vi "MainLoop.vi"() -> ()   [LabVIEW 2021]
uses:
  <vilib>/Platform/TimedLoop/XDataNode/timing_clust.ctl
  <vilib>/Platform/TimedLoop/XDataNode/nitl_modes.ctl
  <vilib>/Platform/TimedLoop/XDataNode/wakeup.ctl
  <vilib>/DAQmx/write.llb/DAQmx Write (Analog 1D DBL NChan 1Samp).vi
  <vilib>/DAQmx/read.llb/DAQmx Read (Analog 1D DBL NChan 1Samp).vi
  5a09477c-fa6a-4a2c-ae4e-0462b0b96a3d.vi
  6f825153-6f78-4197-a3b4-cb3bcc6ce098.vi
  <vilib>/DAQmx/create/channels.llb/DAQmx Create Channel (AO-Voltage-Basic).vi
  <vilib>/DAQmx/create/channels.llb/DAQmx Create Channel (AI-Voltage-Basic).vi
  GlobalSTATE.vi
  <vilib>/DAQmx/miscellaneous.llb/DAQmx Fill In Error Info.vi
  Global_BeamBreaks.vi
  <vilib>/Utility/file.llb/Write Delimited Spreadsheet (string).vi
  <vilib>/Utility/file.llb/Read Delimited Spreadsheet (DBL).vi
  <vilib>/platform/TimedLoop/XDataNode/XDataNode.xnode
  <vilib>/Platform/TimedLoop/XDataNode/XDNodeRunTimeDep.lvlib
panel:
  out "ConditionVoltage":dbl
  out "BeamVoltage":dbl
  in  "stop":bool
  in  "Tab Control":enum32{"Settings", "Monitor", "Events"}(tab)
  in  "Task type":T1(ring)
  in  "Drive to change (in 'One drive changes')":enum32{"Food", "Water", "Social"}(ring)
  in  "Possible availability":i32[](array[numeric])=[0, 1, 2]
  in  "Control availability":i32=1
  in  "Availability settings":i32[][](array[numeric])=[[0, 1, 3], [0, 1, 3], [0, 3000, 9000]]
  in  "file (use dialog)":path=path "C:/Code/Availability-maze-main/Availability-maze-main/MazeCode/LookUpTbl.txt"
  in  "thresholds":dbl[](array[numeric])=[3.0, 2.0, 2.0, 2.0, 2.0, 2.0]
  in  "Beam breaks":bool[](array[boolean])
  out "Current State":string="Condition: l - 210"
  out "Block length":i32=3
  out "Max pellets":u32=2
  out "Interaction time (ms)":u32
  out "Max water drops":u32=1
  out "Block count":i32
  out "Trial of block":i32
  out "Food available":dbl(knob)=2.0 scale=0.0..3.0
  out "Water available":dbl(knob)=1.0 scale=0.0..3.0
  out "Social time available":dbl(knob) scale=0.0..10000.0
  out "serial comm":string="l"
  out "ms in nest":i32
  out "NEST":bool=TRUE
  out "Event times":string[][](array[string])=[["05/06/2022", "14:41:05", "SOCIAL TIME"], ["05/06/2022", "14:41:05", "Condition: l - 210"]]
  in  "Save event file?":bool
  in  "file path (dialog if empty)":path=path "C:/temp/EventData/222"
  # "Social\n\nWater\n\nFood\n\nMiddle 1\n\nMiddle 2\n\nHome cage"
  # "Low (0)     Medium (1)    High(2)"
  # "Pellets \n\nWater drops\n\nSocial time (ms)"
  # "This should stay at 1"
  # "Social                Water                  Food               Middle            Middle 2       Home cage"
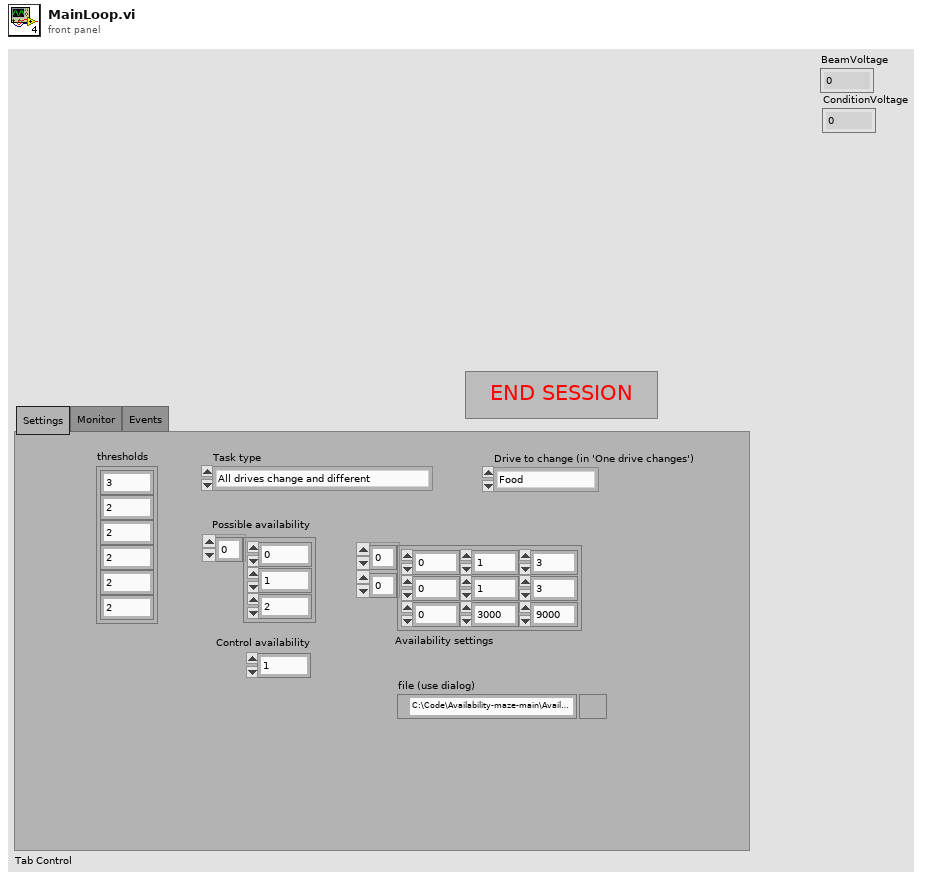
[diagram p1: front panel]
types:
  T1 = enum32{"All drives change and different", "One drive changes", "All drives same, but change"}
  T2 = typedef "XDNodeRunTimeDep.lvlib/timing_clust.ctl" = cluster{"Expected End [f-1]":u64, "Actual End [f-1]":u64, "Finished Late? [f-1]":bool, "Expected End [i-1]":u64, "Actual End [i-1]":u64, "Finished Late? [i-1]":bool, "Expected Start [i]":u64, "Actual Start [i]":u64, "Expected Start [f]":u64, "Actual Start [f]":u64, "Source Name":string, "Structure Name":string, "Period":i64, "Deadline":i64, "Offset":i64, "Start":i64, "Priority":i32, "Timeout":i32, "Mode":T3, "Wakeup Reason":T4, "Error":errorcluster, "Source Type":string, "Secondary Source Type":string, "Global End Time":u64, "Global Start Time":u64, "Frame Duration":u64, "Iteration Duration":u64, "Assigned CPU":i32, "I/O Scan Engine Mode":u32}
  T3 = typedef "XDNodeRunTimeDep.lvlib/nitl_modes.ctl" = enum32{"No Change", "Process missed periods, maintain original phase", "Discard missed periods, maintain original phase", "Process missed periods, ignore original phase", "Discard missed periods, ignore original phase"}
  T4 = typedef "XDNodeRunTimeDep.lvlib/wakeup.ctl" = enum32{"Normal", "Aborted", "Asynchronous wakeup", "Timing source error", "Timed loop error", "Timeout"}
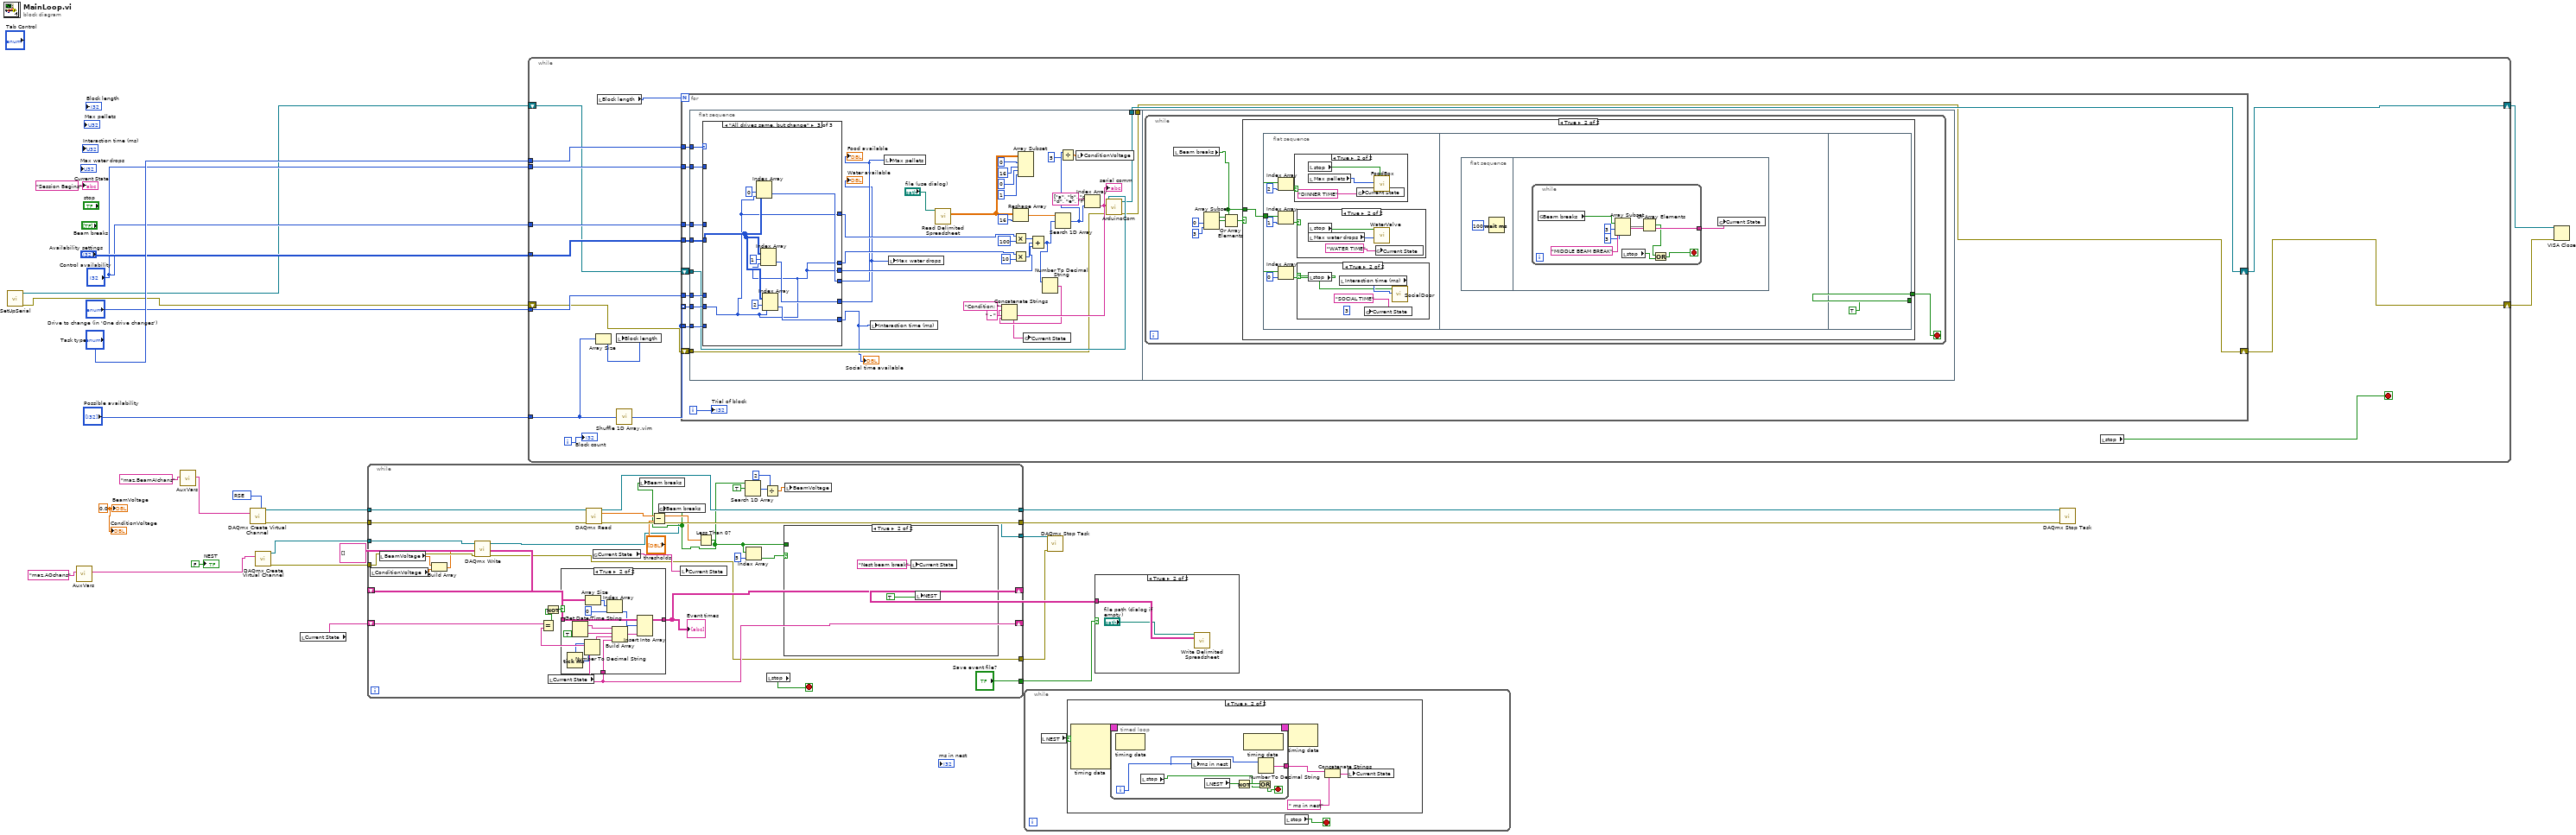
[diagram p0: block diagram]
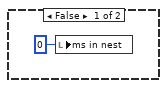
[diagram p2: hidden frame]
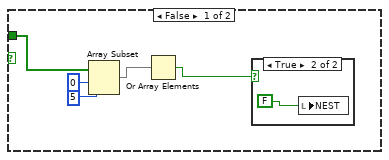
[diagram p4: hidden frame]
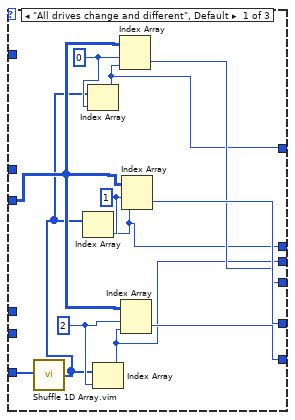
[diagram p7: hidden frame]
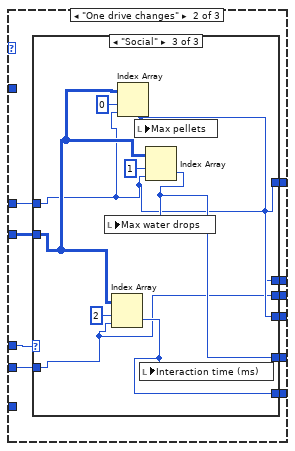
[diagram p8: hidden frame]
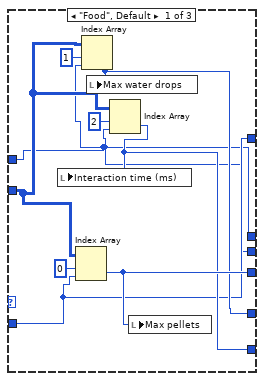
[diagram p9: hidden frame]
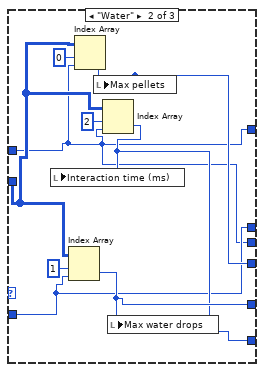
[diagram p10: hidden frame]
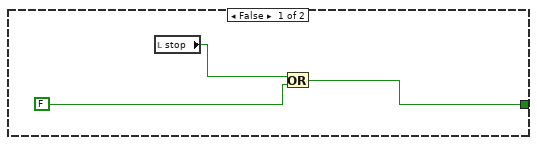
[diagram p11: hidden frame]
diagram:
  w9 = 0.0 ("BeamVoltage")
  w14 = 10083 items=["Default"=-1, "RSE"=10083, "NRSE"=10078, "Differential"=10106, "Pseudodifferential"=12529] ("input terminal configuration")
  n1 = call "SetUpSerial.vi"() -> ("error out"=w1:errorcluster, "VISA resource name out"=w16:refnum<visa-resource-name>)  [unwired: 10 in]
  n2 = call "AuxVars.vi"("key"="maz.AOchans") -> ("value"=w5:string)  [unwired: 9 in, 1 out]
  n3 = call "AuxVars.vi"("key"="maz.BeamAIchans") -> ("value"=w3:string)  [unwired: 9 in, 1 out]
  n4 = call-poly <vilib>:"DAQmx Create Virtual Channel.vi"("input terminal configuration"=w14, "physical channels"=w3) -> ("task out"=w29:refnum<k21>, "error out"=w28:errorcluster)  [unwired: 12 in]
  n5 = call-poly <vilib>:"DAQmx Create Virtual Channel.vi"("physical channels"=w5) -> ("task out"=w11:refnum<k21>, "error out"=w10:errorcluster)  [unwired: 13 in]
  n6 = local read "Current State"() -> (w18:string)
  n7 = while {
    tunnel: w29 -> [w59]
    tunnel: w28 -> [w58]
    tunnel: [w57] -> w27
    tunnel: [w56] -> w26
    shift-right: [w51] -> w17
    shift-left: string[][] [] -> [w52]
    shift-right: [w50] -> _
    shift-left: w18 -> [w49]
    tunnel: ["Save event file?"] -> w13
    tunnel: w11 -> [w41]
    tunnel: w10 -> [w40]
    tunnel: [w31] -> w8
    tunnel: [w30] -> w7
    stop <- w55 stop-if-true
    n8 = local read "ConditionVoltage"() -> (w33:dbl)
    n9 = local read "BeamVoltage"() -> (w34:dbl)
    n10 = Build Array(w34, w33) -> (w32:dbl[])
    n11 = call-poly <vilib>:"DAQmx Write.vi"("task/channels in"=w41, "data"=w32, "error in"=w40) -> ("task out"=w31:refnum<k21>, "error out"=w30:errorcluster)  [unwired: 10 in, 1 out]
    n12 = local read "Current State"() -> (w50:string)
    n13 = Equal?(x=w49, y=w50) -> (x = y?=w53:bool)
    n14 = Not(x=w53) -> (.not. x?=w54:bool)
    n15 = case shown="True" w54 {
      tunnel: w52 -> [w68 w80]
      tunnel: [w68 w79] -> w51
      tunnel: w50 -> [_ w74]
      frame False {
      }
      frame True {
        n16 = Tick Count (ms)() -> (millisecond timer value=w69:u32)
        n17 = Get Date/Time String(want seconds? (F)=TRUE) -> (date string=w73:string, time string=w71:string)  [unwired: 2 in]
        n18 = Number To Decimal String(number=w69, width (-)=w69) -> (decimal integer string=w70:string)
        n19 = Array Size(array=w80) -> (size(s)=w78:i32[])
        n20 = Index Array(array=w78, index=0) -> (element=w76:i32)
        n21 = Build Array(w73, w71, w70, w74) -> (w75:string[])
        n22 = Insert Into Array(array=w80, index (row)=w76, new element=w75) -> (w79:string[][])  [unwired: 1 in]
      }
    }
    "Event times" <- w51
    n23 = call-poly <vilib>:"DAQmx Read.vi"("task/channels in"=w59, "error in"=w58) -> ("task out"=w57:refnum<k21>, "data"=w46:dbl[], "error out"=w56:errorcluster)  [unwired: 11 in]
    n24 = global read "GlobalSTATE.vi" "Current State"() -> (w48:string)
    n25 = Subtract(x=w46, y="thresholds") -> (x-y=w47:dbl[])
    n26 = local write "Current State"(w48) -> ()
    n27 = Less Than 0?(x=w47) -> (x < 0?=w36:bool[])
    n28 = local write "Beam breaks"(w36) -> ()
    n29 = global write "Global_BeamBreaks.vi" "Beam breaks"(w36) -> ()
    n30 = Search 1D Array(1D array=w36, element=TRUE) -> (index of element=w39:i32)  [unwired: 1 in]
    n31 = Index Array(array=w36, index=5) -> (element=w43:bool)
    n32 = Divide(x=w39, y=2) -> (x/y=w37:dbl)
    n33 = local read "stop"() -> (w55:bool)
    n34 = case shown="True" w43 {
      tunnel: w36 -> [w64 _]
      frame False {
        n35 = Array Subset(array=w64, index=0, length=5) -> (w61:bool[])
        n36 = Or Array Elements(Boolean array=w61) -> (logical OR=w60:bool)
        n37 = case shown="True" w60 {
          frame False {
          }
          frame True {
            n38 = local write "NEST"(FALSE) -> ()
          }
        }
      }
      frame True {
        n39 = local write "Current State"("Nest beam break" ("Current State")) -> ()
        n40 = local write "NEST"(TRUE) -> ()
      }
    }
    n41 = local write "BeamVoltage"(w37) -> ()
  }
  n42 = while {
    tunnel: "Task type" -> [w95]
    tunnel: "Drive to change (in 'One drive changes')" -> [w94]
    tunnel: "Possible availability" -> [w89]
    tunnel: "Availability settings" -> [w93]
    tunnel: "Control availability" -> [w92]
    tunnel: "Control availability" -> [w91]
    shift-right: [w82] -> w2
    shift-left: w16 -> [w84]
    shift-right: [w81] -> w15
    shift-left: w1 -> [w83]
    i -> [w87]
    stop <- w85 stop-if-true
    n43 = Array Size(array=w89) -> (size(s)=w88:i32)
    n44 = local read "Block length"() -> (w90:i32)
    n45 = local write "Block length"(w88) -> ()
    n46 = call "Shuffle 1D Array.vim"("array"=w89) -> ("shuffled array"=w86:i32[])  [unwired: 4 in]
    n47 = for {
      N: w90 -> [_]
      tunnel: w95 -> [w107]
      tunnel: w94 -> [w106]
      tunnel: w86 -> [w105] mode=indexing
      tunnel: w93 -> [w104]
      tunnel: w92 -> [w103]
      tunnel: w91 -> [w102]
      tunnel: w86 -> [w100]
      shift-right: [w97] -> w82
      shift-left: w84 -> [w99]
      shift-right: [w96] -> w81
      shift-left: w83 -> [w98]
      i -> [w101]
      n48 = flat-sequence {
        tunnel: w107 -> [w146]
        tunnel: w106 -> [w145]
        tunnel: w105 -> [w144]
        tunnel: w104 -> [w143]
        tunnel: w103 -> [w142]
        tunnel: w102 -> [w141]
        tunnel: w100 -> [w140]
        tunnel: w99 -> [w117]
        tunnel: w98 -> [w116]
        tunnel: [w115] -> w97
        tunnel: [w114] -> w96
        frame #0 {
          n49 = case shown="\"All drives same, but change\"" w146 {
            tunnel: w145 -> [_ w168 _]
            tunnel: w144 -> [_ w167 w196]
            tunnel: w143 -> [w158 w166 w200]
            tunnel: w142 -> [_ _ _]
            tunnel: w141 -> [_ w165 _]
            tunnel: [w150 w164 w199] -> w112
            tunnel: [w151 w163 w198] -> w111
            tunnel: [w155 w162 w197] -> w113
            tunnel: w140 -> [w157 _ _]
            tunnel: [w149 w161 w196] -> w137
            tunnel: [w148 w160 w196] -> w136
            tunnel: [w147 w159 w196] -> w135
            frame "All drives change and different", Default {
              w154 = 0 ("index")
              w153 = 1 ("index")
              w156 = 2 ("index")
              n50 = call "Shuffle 1D Array.vim"("array"=w157) -> ("shuffled array"=w152:i32[])  [unwired: 4 in]
              n51 = Index Array(array=w152, index=w153) -> (element=w148:i32)
              n52 = Index Array(array=w152, index=w154) -> (element=w149:i32)
              n53 = Index Array(array=w152, index=w156) -> (element=w147:i32)
              n54 = Index Array(array=w158, index (row)=w154, index (col)=w149) -> (element=w150:i32)
              n55 = Index Array(array=w158, index (row)=w156, index (col)=w147) -> (element=w155:i32)
              n56 = Index Array(array=w158, index (row)=w153, index (col)=w148) -> (element=w151:i32)
            }
            frame "One drive changes" {
              n57 = case shown="\"Social\"" w168 {
                tunnel: w167 -> [w170 w179 w187]
                tunnel: w166 -> [w174 w183 w192]
                tunnel: w165 -> [w169 w178 w188]
                tunnel: [w173 w182 w189] -> w164
                tunnel: [w172 w181 w191] -> w163
                tunnel: [w171 w180 w190] -> w162
                tunnel: [w170 w178 w188] -> w161
                tunnel: [w169 w179 w188] -> w160
                tunnel: [w169 w178 w187] -> w159
                frame "Food", Default {
                  n58 = Index Array(array=w174, index (row)=0 ("index"), index (col)=w170) -> (element=w173:i32)
                  n59 = Index Array(array=w174, index (row)=1, index (col)=w169) -> (element=w172:i32)
                  n60 = local write "Max water drops"(w172) -> ()
                  n61 = Index Array(array=w174, index (row)=2 ("disabled index (row)"), index (col)=w169) -> (element=w171:i32)
                  n62 = local write "Interaction time (ms)"(w171) -> ()
                  n63 = local write "Max pellets"(w173) -> ()
                }
                frame "Water" {
                  n64 = Index Array(array=w183, index (row)=1 ("index"), index (col)=w179) -> (element=w181:i32)
                  n65 = Index Array(array=w183, index (row)=0, index (col)=w178) -> (element=w182:i32)
                  n66 = local write "Max pellets"(w182) -> ()
                  n67 = Index Array(array=w183, index (row)=2 ("disabled index (row)"), index (col)=w178) -> (element=w180:i32)
                  n68 = local write "Interaction time (ms)"(w180) -> ()
                  n69 = local write "Max water drops"(w181) -> ()
                }
                frame "Social" {
                  n70 = Index Array(array=w192, index (row)=2 ("index"), index (col)=w187) -> (element=w190:i32)
                  n71 = Index Array(array=w192, index (row)=0, index (col)=w188) -> (element=w189:i32)
                  n72 = local write "Max pellets"(w189) -> ()
                  n73 = local write "Interaction time (ms)"(w190) -> ()
                  n74 = Index Array(array=w192, index (row)=1 ("disabled index (row)"), index (col)=w188) -> (element=w191:i32)
                  n75 = local write "Max water drops"(w191) -> ()
                }
              }
            }
            frame "All drives same, but change" {
              n76 = Index Array(array=w200, index (row)=0, index (col)=w196) -> (element=w199:i32)
              n77 = Index Array(array=w200, index (row)=1, index (col)=w196) -> (element=w198:i32)
              n78 = Index Array(array=w200, index (row)=2, index (col)=w196) -> (element=w197:i32)
            }
          }
          "Food available" <- w112
          "Water available" <- w111
          "Social time available" <- w113
          n79 = local write "Interaction time (ms)"(w113) -> ()
          n80 = local write "Max pellets"(w112) -> ()
          n81 = local write "Max water drops"(w111) -> ()
          n82 = call-poly <vilib>:"Read Delimited Spreadsheet.vi"("file path (dialog if empty)"="file (use dialog)") -> ("all rows"=w127:dbl[][])  [unwired: 9 in, 5 out]
          n83 = Reshape Array(w127, 16 ("dimension size")) -> (w126:dbl[])
          n84 = Multiply(x=w137, y=100) -> (x*y=w133:i32)
          n85 = Multiply(x=w136, y=10) -> (x*y=w134:i32)
          n86 = Array Subset(array=w127, index (row)=0 ("index"), length (row)=16 ("length"), index (col)=0 ("index"), length (col)=1 ("length")) -> ()  [unwired: 1 out]
          n87 = Compound Arithmetic op=ADD(w133, w134, w135) -> (w120:i32)
          n88 = Number To Decimal String(number=w120) -> (decimal integer string=w119:string)  [unwired: 1 in]
          n89 = Search 1D Array(1D array=w126, element=w120) -> (index of element=w109:i32)  [unwired: 1 in]
          n90 = Divide(x=w109, y=5) -> (x/y=w110:dbl)
          n91 = local write "ConditionVoltage"(w110) -> ()
          n92 = Index Array(array=string[] ["a", "b", "c", "d", "e", "f", "g", "h", "i", "j", "k", "l", "m", "n", "o"], index=w109) -> (element=w122:string)
          "serial comm" <- w122
          n93 = Concatenate Strings("Condition: " ("string"), w122, " - " ("string"), w119) -> (w118:string)
          n94 = global write "GlobalSTATE.vi" "Current State"(w118) -> ()
          n95 = call "ArduinoCom.vi"("error out"=w116, "write buffer"=w122, "VISA resource name out"=w117) -> ("error out 2"=w114:errorcluster, "VISA resource name out 2"=w115:refnum<visa-resource-name>)  [unwired: 7 in]
        }
        frame #1 {
          n96 = while {
            stop <- w204 stop-if-true
            n97 = local read "Beam breaks"() -> (w205:bool[])
            n98 = Array Subset(array=w205, index=0, length=3) -> (w208:bool[])
            n99 = Or Array Elements(Boolean array=w208) -> (logical OR=w209:bool)
            n100 = case shown="True" w209 {
              tunnel: w205 -> [_ w214]
              tunnel: [w210 w213] -> w204
              frame False {
                n101 = local read "stop"() -> (w211:bool)
                n102 = Or(x=w211, y=FALSE ("stop")) -> (x .or. y?=w210:bool)
              }
              frame True {
                n103 = flat-sequence {
                  tunnel: w214 -> [w215]
                  tunnel: [TRUE ("stop")] -> w213
                  frame #0 {
                    n104 = Index Array(array=w215, index=2) -> (element=w220:bool)
                    n105 = Index Array(array=w215, index=1) -> (element=w216:bool)
                    n106 = Index Array(array=w215, index=0) -> (element=w218:bool)
                    n107 = case shown="True" w220 {
                      frame False {
                      }
                      frame True {
                        n108 = local read "stop"() -> (w228:bool)
                        n109 = local read "Max pellets"() -> (w230:u32)
                        n110 = global write "GlobalSTATE.vi" "Current State"("DINNER TIME" ("Current State")) -> ()
                        n111 = call "FoodBox.vi"("STOP"=w228, "Max pellets"=w230) -> ()  [unwired: 9 in, 1 out]
                      }
                    }
                    n112 = case shown="True" w216 {
                      frame False {
                      }
                      frame True {
                        n113 = local read "stop"() -> (w222:bool)
                        n114 = local read "Max water drops"() -> (w224:u32)
                        n115 = call "WaterValve.vi"("Max pulses"=w224, "STOP"=w222) -> ()  [unwired: 10 in]
                        n116 = global write "GlobalSTATE.vi" "Current State"("WATER TIME" ("Current State")) -> ()
                      }
                    }
                    n117 = case shown="True" w218 {
                      frame False {
                      }
                      frame True {
                        (unwired) 3 ("index")
                        n118 = local read "stop"() -> (w225:bool)
                        n119 = local read "Interaction time (ms)"() -> (w227:u32)
                        n120 = global write "GlobalSTATE.vi" "Current State"("SOCIAL TIME" ("Current State")) -> ()
                        n121 = call "SocialDoor.vi"("Interaction time"=w227, "STOP"=w225) -> ()  [unwired: 10 in]
                      }
                    }
                  }
                  frame #1 {
                    n122 = flat-sequence {
                      frame #0 {
                        n123 = Wait (ms)(milliseconds to wait=u32 100) -> ()  [unwired: 1 out]
                      }
                      frame #1 {
                        n124 = while {
                          tunnel: ["MIDDLE BEAM BREAK" ("Current State")] -> w232
                          stop <- w238 stop-if-true
                          n125 = global read "Global_BeamBreaks.vi" "Beam breaks"() -> (w235:bool[])
                          n126 = Array Subset(array=w235, index=3, length=3) -> (w234:bool[])
                          n127 = local read "stop"() -> (w239:bool)
                          n128 = Or Array Elements(Boolean array=w234) -> (logical OR=w233:bool)
                          n129 = Or(x=w233, y=w239) -> (x .or. y?=w238:bool)
                        }
                        n130 = global write "GlobalSTATE.vi" "Current State"(w232) -> ()
                      }
                    }
                  }
                  frame #2 {
                  }
                }
              }
            }
          }
        }
      }
      "Trial of block" <- w101
    }
    n131 = local read "stop"() -> (w85:bool)
    "Block count" <- w87
  }
  n132 = while {
    stop <- w242 stop-if-true
    n133 = local read "NEST"() -> (w243:bool)
    n134 = case shown="True" w243 {
      frame False {
        n135 = local write "ms in nest"(0 ("ms in nest")) -> ()
      }
      frame True {
        n136 = node-c288() -> (w249:T2)  [unwired: 4 in]
        n137 = timed-loop {
          timing: w249 -> [_]
          timing-out: [_] -> w248
          tunnel: [w253] -> w247
          i -> [w254]
          stop <- w250 stop-if-true
          n138 = node-c288() -> ()  [unwired: 1 in, 1 out]
          n139 = local read "stop"() -> (w251:bool)
          n140 = local write "ms in nest"(w254) -> ()
          n141 = local read "NEST"() -> (w255:bool)
          n142 = Not(x=w255) -> (.not. x?=w252:bool)
          n143 = node-c288() -> ()  [unwired: 1 in, 1 out]
          n144 = Or(x=w252, y=w251) -> (x .or. y?=w250:bool)
          n145 = Number To Decimal String(number=w254) -> (decimal integer string=w253:string)  [unwired: 1 in]
        }
        n146 = node-c288(w248) -> ()  [unwired: 1 out]
        n147 = Concatenate Strings(w247, " ms in nest" ("string")) -> (w245:string)
        n148 = local write "Current State"(w245) -> ()
      }
    }
    n149 = local read "stop"() -> (w242:bool)
  }
  n150 = call <vilib>:"DAQmx Stop Task.vi"("task/channels in"=w8, "error in"=w7) -> ()  [unwired: 12 in, 2 out]
  n151 = case shown="True" w13 {
    tunnel: w17 -> [_ w261]
    frame False {
    }
    frame True {
      n152 = call-poly <vilib>:"Write Delimited Spreadsheet.vi"("file path (dialog if empty)"="file path (dialog if empty)", "2D data"=w261) -> ()  [unwired: 12 in, 2 out]
    }
  }
  n153 = call <vilib>:"DAQmx Stop Task.vi"("task/channels in"=w27, "error in"=w26) -> ()  [unwired: 12 in, 2 out]
  n154 = VISA Close(VISA resource name=w2, error in (no error)=w15) -> ()  [unwired: 1 out]
  "Current State" <- "Session Begins" ("Current State")
  "NEST" <- FALSE ("NEST")
  "BeamVoltage" <- w9
  "ConditionVoltage" <- w9
